vi "AlliGator Formula Interpreter.vi"(8 "error in (no error)":errorcluster, 11 "Original Formula":string) -> (0 "error out":errorcluster, 1 "Variable Names":cluster{"Array of Names":string[]}, 2 "Variable Indices":cluster{"Array of Indices":i32[]}, 3 "Interpreted Formula":string, 4 "Unused Flag":bool)   [LabVIEW 2021, in "AlliGator Phasor Plot.lvlib"]
doc: "Replaces user quantities by definitions in the provided formula."
uses:
  AlliGator Phasor Plot.lvlib
  Formula/Formula.lvlib
panel:
  # "see the AlliGator License on the block diagram (Ctrl+E or Window:Show Block Diagram)"
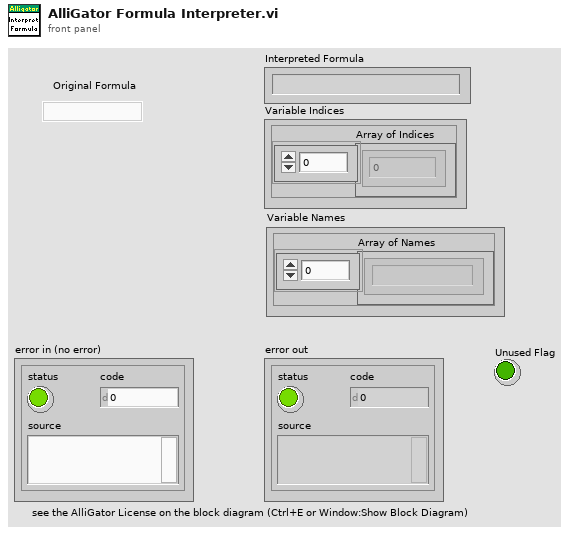
[diagram p1: front panel]
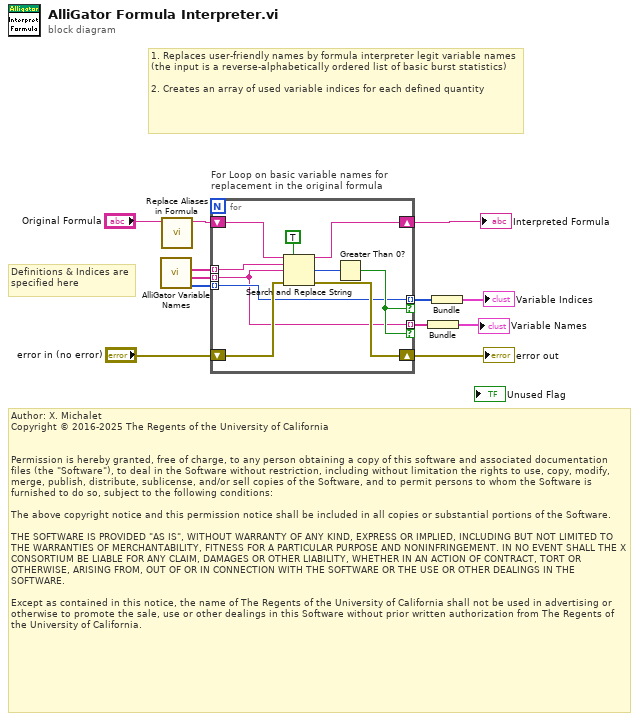
[diagram p0: block diagram]
diagram:
  # "Author: X. Michalet\nCopyright © 2016-2025 The Regents of the University of California\n \n\nPermission is hereby granted, free of charge, to any person obtaining a copy of this software and associated documentation files (the \"Software\"), to deal in the Software without restriction, including without limitation the rights to use, copy, modify, merge, publish, distribute, sublicense, and/or sell copies of the Software, and to permit persons to whom the Software is furnished to do so, subject to the following conditions:\n\nThe above copyright notice and this permission notice shall be included in all copies or substantial portions of the Software.\n\nTHE SOFTWARE IS PROVIDED \"AS IS\", WITHOUT WARRANTY OF ANY KIND, EXPRESS OR IMPLIED, INCLUDING BUT NOT LIMITED TO THE WARRANTIES OF MERCHANTABILITY, FITNESS FOR A PARTICULAR PURPOSE AND NONINFRINGEMENT. IN NO EVENT SHALL THE X CONSORTIUM BE LIABLE FOR ANY CLAIM, DAMAGES OR OTHER LIABILITY, WHETHER IN AN ACTION OF CONTRACT, TORT OR OTHERWISE, ARISING FROM, OUT OF OR IN CONNECTION WITH THE SOFTWARE OR THE USE OR OTHER DEALINGS IN THE SOFTWARE.\n\nExcept as contained in this notice, the name of The Regents of the University of California shall not be used in advertising or otherwise to promote the sale, use or other dealings in this Software without prior written authorization from The Regents of the University of California."
  # "Definitions & Indices are specified here"
  # "1. Replaces user-friendly names by formula interpreter legit variable names (the input is a reverse-alphabetically ordered list of basic burst statistics)\n\n2. Creates an array of used variable indices for each defined quantity"
  n1 = call "AlliGator Variable Names.vi"() -> ("Sorted Index Array"=w1:i32[], "Sorted Variable Internal Names"=w2:string[], "Sorted Basic Variable Names"=w3:string[])  [unwired: 5 in, 1 out]
  n2 = call "Replace Aliases in Formula.vi"("Definition in"="Original Formula") -> ("Expanded Definition out"=w4:string)  [unwired: 10 in]
  n3 = for "For Loop on basic variable names for replacement in the original formula" {
    tunnel: w3 -> [w21] mode=indexing
    shift-right: [w20] -> w8
    shift-left: w4 -> [w22]
    shift-right: [w18] -> w10
    shift-left: "error in (no error)" -> [w19]
    tunnel: [w14] -> w11 mode=indexing if=w15
    tunnel: [w13] -> w7 mode=indexing if=w15
    tunnel: w2 -> [w13] mode=indexing
    tunnel: w1 -> [w14] mode=indexing
    n4 = Search and Replace String(replace all?=TRUE ("replace all? (F)"), input string=w22, search string=w21, replace string=w13, error in=w19) -> (result string=w20:string, number of replacements=w17:i32, error out=w18:errorcluster)  [unwired: 3 in, 1 out]
    n5 = Greater Than 0?(x=w17) -> (x > 0?=w15:bool)
  }
  "error out" <- w10
  "Interpreted Formula" <- w8
  n6 = Bundle(w7) -> (→"Variable Names":cluster{string[]})  [unwired: 1 in]
  n7 = Bundle(w11) -> (→"Variable Indices":cluster{i32[]})  [unwired: 1 in]
